vi "DatabaseSearching.vi"(0 "Account Details":T1[](array[typedef])=[{"Card Number"=1.0, "Card Holder Name"="Selva Gowtham", "Valid Upto"=34.0}, {"Card Number"=2.0, "Card Holder Name"="Puviyarasu", "Valid Upto"=32.0}, {"Card Number"=3.0, "Card Holder Name"="Krishnan", "Valid Upto"=23.0}, {"Card Number"=4.0, "Card Holder Name"="Mohan Kumar", "Valid Upto"=34.0}], 5 "Search Option":T2, 7 "Card Holder Name":string, 9 "Card Number":dbl, 11 "Valid Upto":dbl) -> (4 "Card Holder Name Search Result":T1[](array[typedef]), 6 "Card Number Search Result":T1, 8 "Valid Upto Search Result":T1[](array[typedef]))   [LabVIEW 2020]
uses:
  Typedefs/AccountDetails.ctl
  Typedefs/CaseSelecting.ctl
panel:
  in  "Stop":bool
  # "Database"
  # "Search Options"
  # "First populate the database values. Then select the criteria from search from the Search Options.\nThen enter the values to be searched. The search results will be displayed."
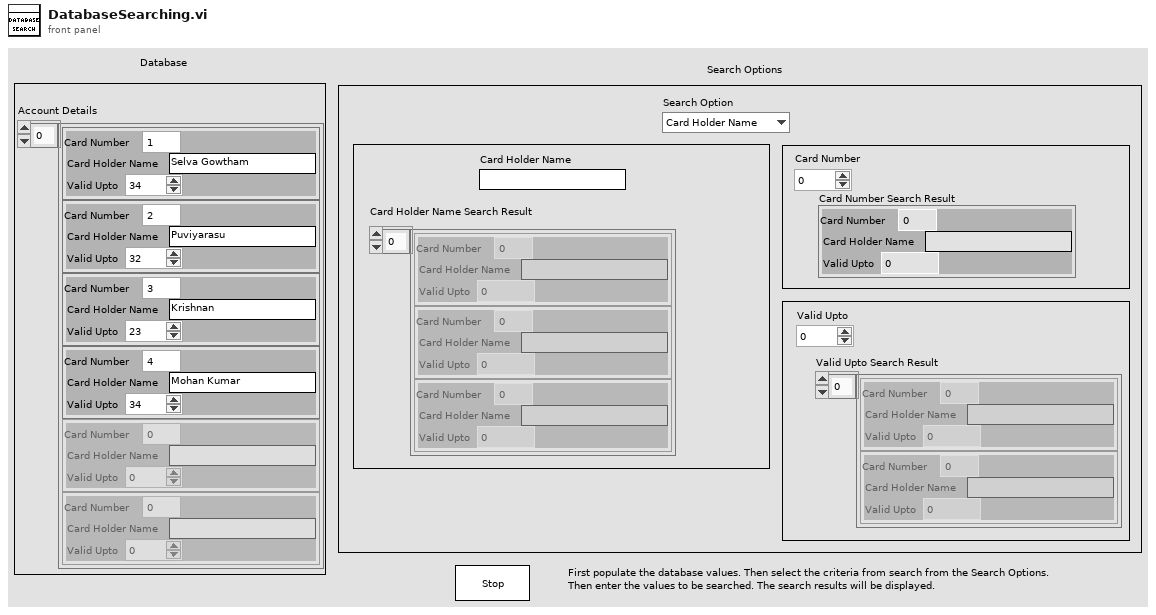
[diagram p1: front panel]
types:
  T1 = typedef "AccountDetails.ctl" = cluster{"Card Number":dbl, "Card Holder Name":string, "Valid Upto":dbl}
  T2 = typedef "CaseSelecting.ctl" = enum16{"Card Holder Name", "Card Number", "Valid upto"}
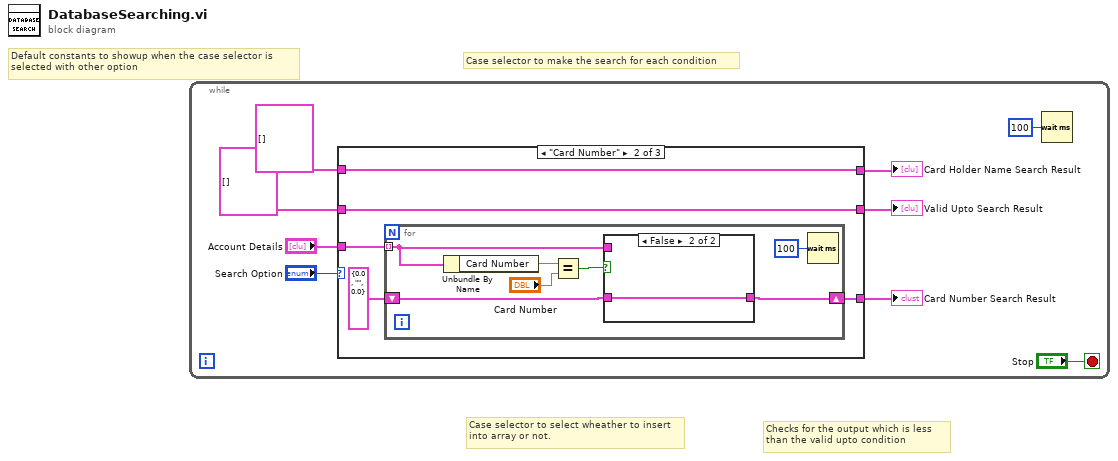
[diagram p0: block diagram]
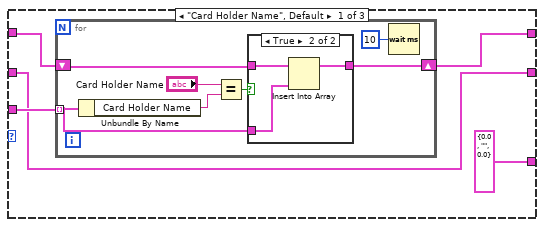
[diagram p2: hidden frame]
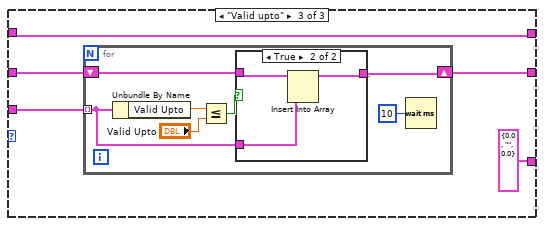
[diagram p5: hidden frame]
diagram:
  # "Checks for the output which is less\nthan the valid upto condition"
  # "Default constants to showup when the case selector is \nselected with other option"
  # "Case selector to select wheather to insert\ninto array or not."
  # "Case selector to make the search for each condition"
  n1 = while {
    stop <- "Stop" stop-if-true
    n2 = case shown="\"Card Number\"" "Search Option" {
      tunnel: T1[] [] ("Array") -> [w10 w30 w44]
      tunnel: [w14 w30 w44] -> w8
      tunnel: "Account Details" -> [w13 w29 w42]
      tunnel: T1[] [] ("Array") -> [w12 w28 w43]
      tunnel: [w12 w28 w41] -> w4
      tunnel: [T1 {"Card Number"=0.0, "Card Holder Name"="", "Valid Upto"=0.0} ("Cluster") w27 T1 {"Card Number"=0.0, "Card Holder Name"="", "Valid Upto"=0.0} ("Cluster")] -> w3
      frame "Card Holder Name", Default {
        n3 = for {
          tunnel: w13 -> [w17] mode=indexing
          shift-right: [w18] -> w14
          shift-left: w10 -> [w19]
          n4 = Unbundle By Name(w17) -> ("Card Holder Name"=w15:string)
          n5 = Equal?(x="Card Holder Name", y=w15) -> (x = y?=w20:bool)
          n6 = case shown="True" w20 {
            tunnel: w17 -> [_ w23]
            tunnel: w19 -> [w22 w25]
            tunnel: [w22 w24] -> w18
            frame False {
            }
            frame True {
              n7 = Insert Into Array(array=w25, new element=w23) -> (w24:T1[])  [unwired: 1 in]
            }
          }
          n8 = Wait (ms)(milliseconds to wait=u32 10) -> ()  [unwired: 1 out]
        }
      }
      frame "Card Number" {
        n9 = for {
          tunnel: w29 -> [w35] mode=indexing
          shift-right: [w34] -> w27
          shift-left: T1 {"Card Number"=0.0, "Card Holder Name"="", "Valid Upto"=0.0} ("Cluster") -> [w31]
          n10 = Unbundle By Name(w35) -> ("Card Number"=w37:dbl)
          n11 = Equal?(x=w37, y="Card Number") -> (x = y?=w33:bool)
          n12 = case shown="False" w33 {
            tunnel: w35 -> [w38 _]
            tunnel: [w38 w39] -> w34
            tunnel: w31 -> [_ w39]
            frame True {
            }
            frame False {
            }
          }
          n13 = Wait (ms)(milliseconds to wait=u32 100) -> ()  [unwired: 1 out]
        }
      }
      frame "Valid upto" {
        n14 = for {
          shift-right: [w49] -> w41
          shift-left: w43 -> [w51]
          tunnel: w42 -> [w50] mode=indexing
          n15 = Unbundle By Name(w50) -> ("Valid Upto"=w47:dbl)
          n16 = Less Or Equal?(x=w47, y="Valid Upto") -> (x <= y?=w48:bool)
          n17 = case shown="True" w48 {
            tunnel: w51 -> [w52 w55]
            tunnel: w50 -> [_ w54]
            tunnel: [w52 w53] -> w49
            frame False {
            }
            frame True {
              n18 = Insert Into Array(array=w55, new element=w54) -> (w53:T1[])  [unwired: 1 in]
            }
          }
          n19 = Wait (ms)(milliseconds to wait=u32 10) -> ()  [unwired: 1 out]
        }
      }
    }
    "Card Holder Name Search Result" <- w8
    "Valid Upto Search Result" <- w4
    "Card Number Search Result" <- w3
    n20 = Wait (ms)(milliseconds to wait=u32 100) -> ()  [unwired: 1 out]
  }
